vi "Set Attribute.vi"(7 "Tree ID":string, 8 "Error In":errorcluster, 9 "Attribute Value":variant, 10 "Attribute Name":string, 11 "Tree Manager":T1) -> (0 "Error Out":errorcluster, 2 "Replaced?":bool, 3 "Tree Manager":T1)   [LabVIEW 2020, in "NI_VIAnCFGDataStructure.lvlib" / "Tree.lvclass"]
doc: "Set a variant data as an attribute of the Tree."
uses:
  <vilib>/addons/analyzer/VIAnCFGDataStructure/Tree Manager/Tree.lvclass
  <vilib>/addons/analyzer/VIAnCFGDataStructure/Tree Manager/Typedefs/Session Handle.ctl
  <vilib>/addons/analyzer/VIAnCFGDataStructure/Tree Manager/Tree.lvclass/Tree.ctl
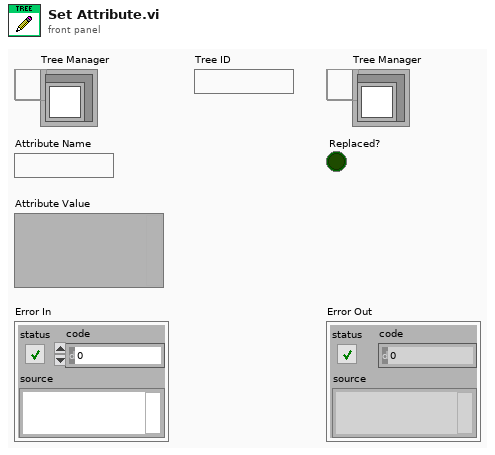
[diagram p1: front panel]
types:
  T1 = typedef "NI_VIAnCFGDataStructure.lvlib/Tree.lvclass/Session Handle.ctl" = refnum<data-value>
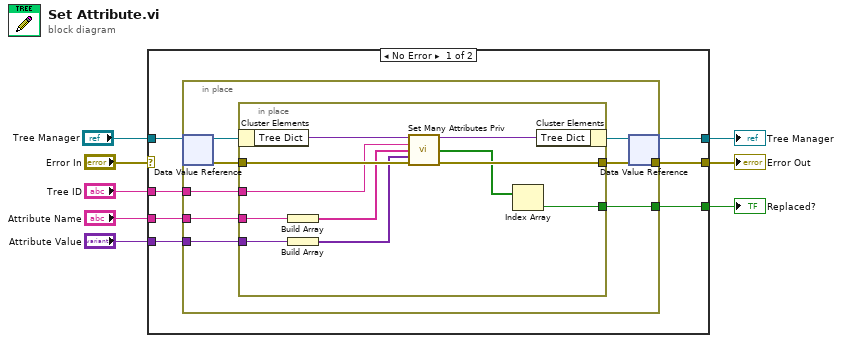
[diagram p0: block diagram]
diagram:
  n1 = case shown="No Error" "Error In" {
    selector: "Error In" -> [_ w35]
    tunnel: "Tree Manager" -> [w10 w36]
    tunnel: [w9 w36] -> w1
    tunnel: [w15 w35] -> w7
    tunnel: "Tree ID" -> [w14 _]
    tunnel: "Attribute Value" -> [w13 _]
    tunnel: "Attribute Name" -> [w12 _]
    tunnel: [w11 _] -> w3
    frame No Error {
      n2 = in-place {
        in-place-border: [w23] -> w15
        in-place-border: w14 -> [w22]
        in-place-border: w13 -> [w21]
        in-place-border: w12 -> [w20]
        in-place-border: [w19] -> w11
        n3 = in-place-dvr #1(w10) -> (w17:refnum<class "Tree.lvclass">, w18:errorcluster)
        n4 = in-place {
          in-place-border: [w26] -> w23
          in-place-border: w18 -> [w32]
          in-place-border: w22 -> [w27]
          in-place-border: w21 -> [w34]
          in-place-border: w20 -> [w33]
          in-place-border: [w24] -> w19
          n5 = in-place-cluster #2(w17) -> ("Tree Dict"=w31:variant)
          n6 = Build Array(w33) -> (w28:string[])
          n7 = Build Array(w34) -> (w29:variant[])
          n8 = call <vilib>:"Set Many Attributes Priv.vi"("Tree Dictionary Out"=w31, "Unique ID"=w27, "Name"=w28, "Data"=w29, "error in"=w32) -> ("Tree Dictionary Out"=w30:variant, "Replaced?"=w25:bool[], "error out"=w26:errorcluster)  [unwired: 8 in]
          n9 = Index Array(array=w25) -> (element=w24:bool)  [unwired: 1 in]
          n10 = in-place-cluster #2("Tree Dict"=w30) -> (w16:refnum<class "Tree.lvclass">)
        }
        n11 = in-place-dvr #1(w16) -> (w9:T1)  [unwired: 1 out]
      }
    }
    frame Error {
    }
  }
  "Error Out" <- w7
  "Replaced?" <- w3
  "Tree Manager" <- w1
